vi "ExtendDevStatus.vi"(8 "offset (0)":i32, 11 "string":string) -> (3 "cluster":T1)   [LabVIEW 2014]
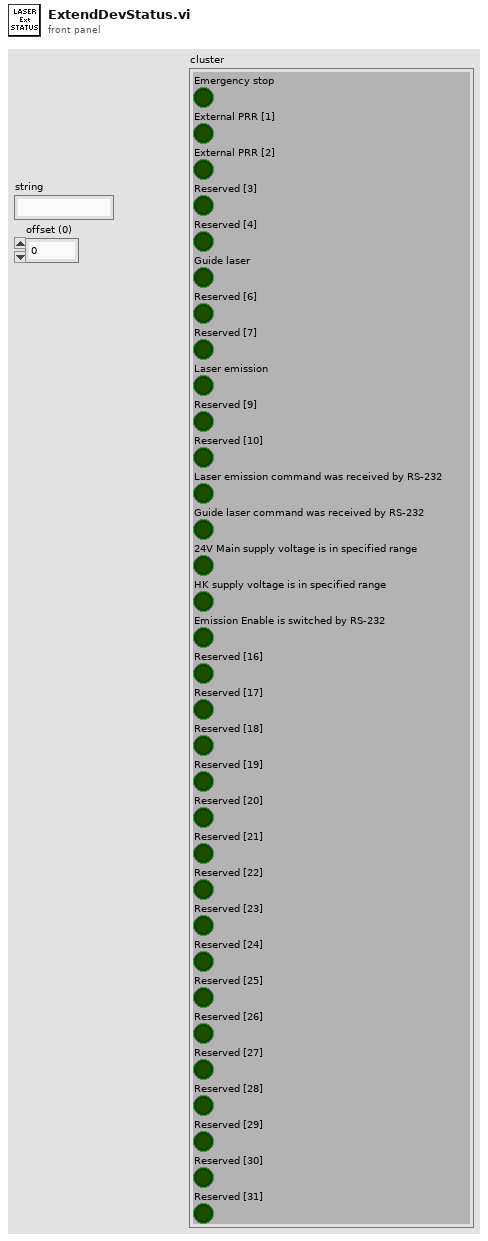
[diagram p1: front panel]
types:
  T1 = cluster{"Emergency stop":bool, "External PRR [1]":bool, "External PRR [2]":bool, "Reserved [3]":bool, "Reserved [4]":bool, "Guide laser":bool, "Reserved [6]":bool, "Reserved [7]":bool, "Laser emission":bool, "Reserved [9]":bool, "Reserved [10]":bool, "Laser emission command was received by RS-232":bool, "Guide laser command was received by RS-232":bool, "24V Main supply voltage is in specified range":bool, "HK supply voltage is in specified range":bool, "Emission Enable is switched by RS-232":bool, "Reserved [16]":bool, "Reserved [17]":bool, "Reserved [18]":bool, "Reserved [19]":bool, "Reserved [20]":bool, "Reserved [21]":bool, "Reserved [22]":bool, "Reserved [23]":bool, "Reserved [24]":bool, "Reserved [25]":bool, "Reserved [26]":bool, "Reserved [27]":bool, "Reserved [28]":bool, "Reserved [29]":bool, "Reserved [30]":bool, "Reserved [31]":bool}
  T2 = cluster{"Boolean array[0]":bool, "Boolean array[1]":bool, "Boolean array[2]":bool, "Boolean array[3]":bool, "Boolean array[4]":bool, "Boolean array[5]":bool, "Boolean array[6]":bool, "Boolean array[7]":bool, "Boolean array[8]":bool, "Boolean array[9]":bool, "Boolean array[10]":bool, "Boolean array[11]":bool, "Boolean array[12]":bool, "Boolean array[13]":bool, "Boolean array[14]":bool, "Boolean array[15]":bool, "Boolean array[16]":bool, "Boolean array[17]":bool, "Boolean array[18]":bool, "Boolean array[19]":bool, "Boolean array[20]":bool, "Boolean array[21]":bool, "Boolean array[22]":bool, "Boolean array[23]":bool, "Boolean array[24]":bool, "Boolean array[25]":bool, "Boolean array[26]":bool, "Boolean array[27]":bool, "Boolean array[28]":bool, "Boolean array[29]":bool, "Boolean array[30]":bool, "Boolean array[31]":bool}
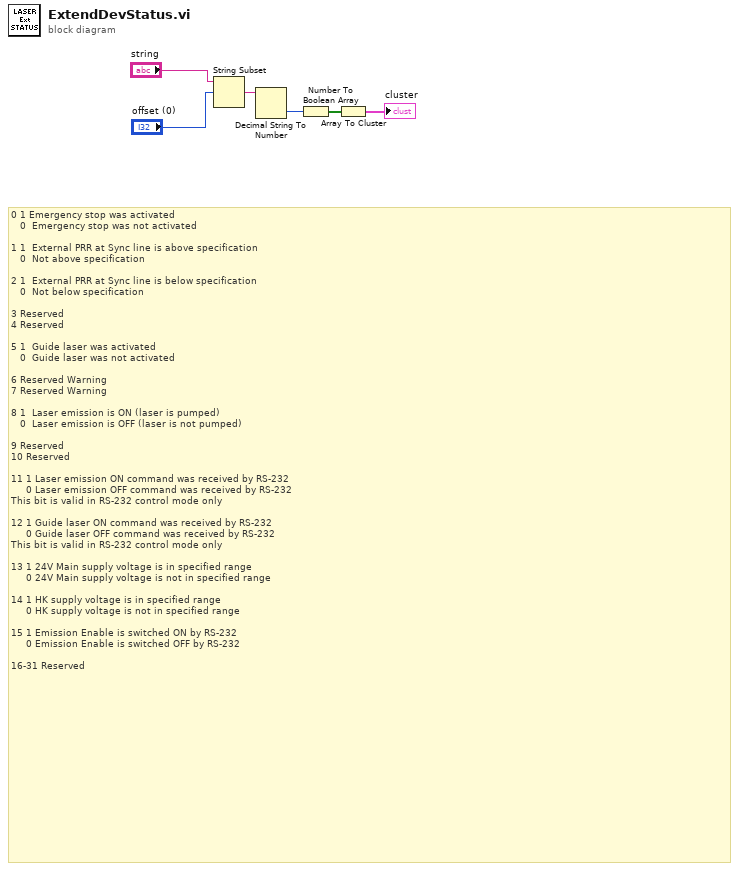
[diagram p0: block diagram]
diagram:
  # "0 1 Emergency stop was activated\n   0  Emergency stop was not activated\n\n1 1  External PRR at Sync line is above specification\n   0  Not above specification\n\n2 1  External PRR at Sync line is below specification\n   0  Not below specification\n\n3 Reserved\n4 Reserved\n\n5 1  Guide laser was activated\n   0  Guide laser was not activated\n\n6 Reserved Warning\n7 Reserved Warning\n\n8 1  Laser emission is ON (laser is pumped)\n   0  Laser emission is OFF (laser is not pumped) \n\n9 Reserved\n10 Reserved\n\n11 1 Laser emission ON command was received by RS-232\n     0 Laser emission OFF command was received by RS-232\nThis bit is valid in RS-232 control mode only\n\n12 1 Guide laser ON command was received by RS-232\n     0 Guide laser OFF command was received by RS-232\nThis bit is valid in RS-232 control mode only\n\n13 1 24V Main supply voltage is in specified range\n     0 24V Main supply voltage is not in specified range\n\n14 1 HK supply voltage is in specified range\n     0 HK supply voltage is not in specified range\n\n15 1 Emission Enable is switched ON by RS-232\n     0 Emission Enable is switched OFF by RS-232\n\n16-31 Reserved"
  n1 = String Subset(string="string", offset (0)="offset (0)") -> (substring=w6:string)  [unwired: 1 in]
  n2 = Decimal String To Number(string=w6) -> (number=w4:i32)  [unwired: 2 in, 1 out]
  n3 = Number To Boolean Array(number=w4) -> (Boolean array=w3:bool[])
  n4 = Array To Cluster(array=w3) -> (cluster=→"cluster":T2)
